vi "dataset.update_add_label.vi"(8 "error in":errorcluster, 11 "DatasetUpdateStaging in":refnum<class "DatasetUpdateStaging.lvclass">) -> (0 "error out":errorcluster, 3 "DatasetUpdateStaging out":refnum<class "DatasetUpdateStaging.lvclass">)   [LabVIEW 2020, in "DatasetUpdateStaging.lvclass"]
doc: "Adds a label to the dataset update being staged, replacing the dataset's entire label set on commit."
uses:
  DatasetUpdateStaging.lvclass
  DatasetUpdateStaging.lvclass/DatasetUpdateStaging.ctl
  client.lvlib
panel:
  in  "label":string
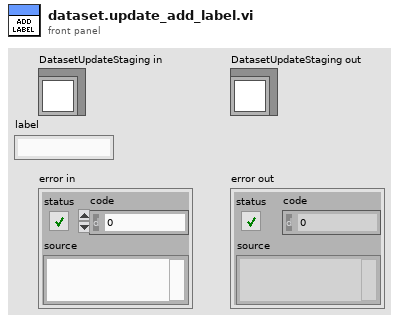
[diagram p1: front panel]
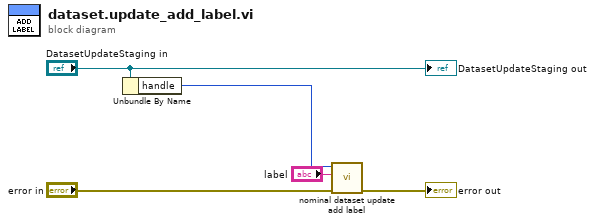
[diagram p0: block diagram]
diagram:
  n1 = Unbundle By Name("DatasetUpdateStaging in") -> ("handle"=w3:i32)
  n2 = call "nominal dataset update add label.vi"("error in (no error)"="error in", "label"="label", "staging"=w3) -> ("error out"=→"error out":errorcluster)  [unwired: 7 in, 1 out]
  "DatasetUpdateStaging out" <- "DatasetUpdateStaging in"
